vi "trial Main.vi"() -> ()   [LabVIEW 2018]
panel:
  out "connecting":bool
  out "sent":bool
  in  "Message":string
  in  "Send":bool
  in  "Quit":bool
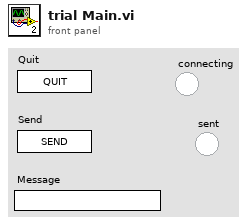
[diagram p1: front panel]
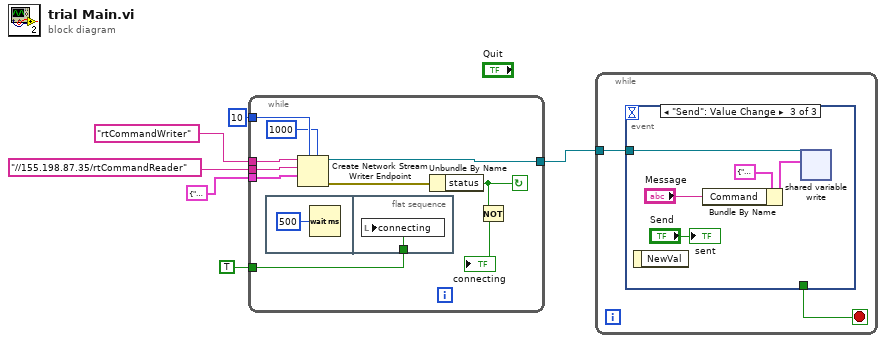
[diagram p0: block diagram]
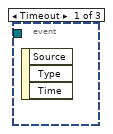
[diagram p2: hidden frame]
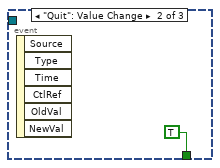
[diagram p3: hidden frame]
diagram:
  n1 = while {
    tunnel: "rtCommandWriter" ("writer name") -> [w16]
    tunnel: cluster{"Command":string, "Data":variant} {"Command"="", "Data"=variant} -> [w15]
    tunnel: "//155.198.87.35/rtCommandReader" ("reader url") -> [w14]
    tunnel: 10 ("writer buffer size") -> [w13]
    tunnel: [w12] -> w2
    tunnel: TRUE ("connecting") -> [w7]
    stop <- w9 continue-if-true
    n2 = flat-sequence {
      tunnel: w7 -> [w18]
      frame #0 {
        n3 = Wait (ms)(milliseconds to wait=u32 500) -> ()  [unwired: 1 out]
      }
      frame #1 {
        n4 = local write "connecting"(w18) -> ()
      }
    }
    n5 = Create Network Stream Writer Endpoint(5:1000 ("timeout in ms (-1)"), 7:w13, 9:w15, 10:w14, 11:w16) -> (0:w11:errorcluster, 3:w12:refnum<k21>)  [unwired: 2 in]
    n6 = Unbundle By Name(w11) -> ("status"=w9:bool)
    n7 = Not(x=w9) -> (.not. x?=→"connecting":bool)
  }
  n8 = while {
    tunnel: w2 -> [w19]
    stop <- w20 stop-if-true
    n9 = event shown="[2] \"Send\": Value Change" {
      selector: _ -> [_ _ _]
      dyn-events: _ -> [_ _ _]
      timeout: _ -> [_ _ _]
      tunnel: [_ TRUE _] -> w20
      tunnel: w19 -> [_ _ w25]
      event Timeout {
        n10 = event-data() -> ()  [unwired: 1 in, 3 out]
      }
      event "Quit": Value Change {
        n11 = event-data() -> ()  [unwired: 1 in, 6 out]
      }
      event "Send": Value Change {
        n12 = event-data() -> ()  [unwired: 1 in, 1 out]
        n13 = Bundle By Name(cluster=cluster{"Command":string, "Data":variant} {"Command"="", "Data"=variant} ("data in"), "Command"="Message") -> (w23:cluster{"Command":string, "Data":variant})
        n14 = shared-variable-write(w25, w23) -> ()  [unwired: 2 in, 3 out]
        "sent" <- "Send"
      }
    }
  }
